vi "DSF Config File to Engine Config Cluster.vi"(8 "error in (no error)":errorcluster, 11 "dsf configuration file path":path) -> (0 "error out":errorcluster, 3 "output cluster":T1)   [LabVIEW 2017, in "Data Sharing Framework Engine.lvlib"]
uses:
  Data Sharing Framework Engine.lvlib
  Configuration/1.0.0/Public/Controls/DSF Engine Framework Configuration.ctl
  Configuration/1.0.0/Public/Controls/DSF Engine Plugin Configuration.ctl
  Configuration/1.0.0/Public/Controls/DSF Timing Info.ctl
  Configuration/1.0.0/Public/Controls/DSF Engine Transfer Group Configuration.ctl
  Configuration/1.0.0/Public/Controls/DSF Direction.ctl
  Configuration/1.0.0/Public/Controls/DSF Engine Transfer Configuration.ctl
  Configuration/1.0.0/Public/Controls/DSF Byte Order.ctl
  Configuration/1.0.0/Public/Controls/DSF Engine Channel Configuration.ctl
  Configuration/1.0.0/Public/Controls/DSF Data Type.ctl
  Configuration/1.0.0/Public/Controls/DSF Settings Info.ctl
  Configuration/1.0.0/Public/Read All Item IDs/Read All Plugin IDs.vi
  Configuration/1.0.0/Public/Read Item/Read Plugin.vi
  Configuration/1.0.0/Public/Read Item/Read Settings.vi
  Configuration/1.0.0/Public/Read Item/Read Group.vi
  Configuration/1.0.0/Public/Read Item/Read Transfer.vi
  Configuration/1.0.0/Public/Read Item/Read Channel.vi
  Configuration/1.0.0/Data Sharing Framework Configuration.lvlib
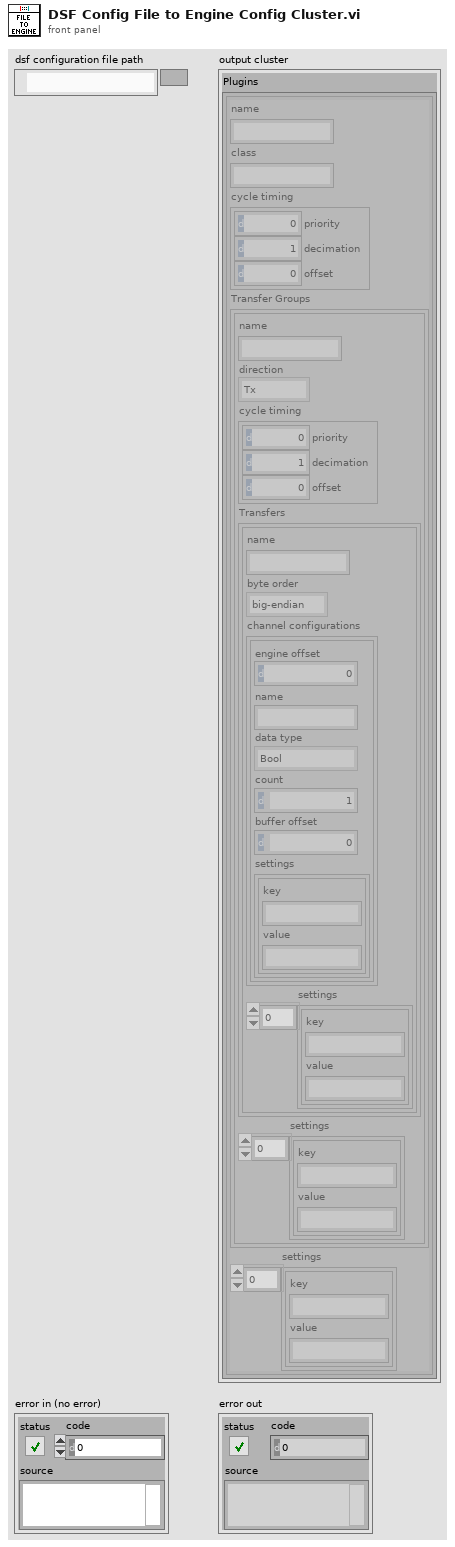
[diagram p1: front panel]
types:
  T1 = typedef "Data Sharing Framework Configuration.lvlib/DSF Engine Framework Configuration.ctl" = cluster{"Plugins":T2[]}
  T2 = typedef "Data Sharing Framework Configuration.lvlib/DSF Engine Plugin Configuration.ctl" = cluster{"name":string, "class":string, "cycle timing":T3, "Transfer Groups":T4[], "settings":T10}
  T3 = typedef "Data Sharing Framework Configuration.lvlib/DSF Timing Info.ctl" = cluster{"priority":u64, "decimation":u64, "offset":u64}
  T4 = typedef "Data Sharing Framework Configuration.lvlib/DSF Engine Transfer Group Configuration.ctl" = cluster{"name":string, "direction":T5, "cycle timing":T3, "Transfers":T6[], "settings":T10}
  T5 = typedef "Data Sharing Framework Configuration.lvlib/DSF Direction.ctl" = enum8{"Tx", "Rx"}
  T6 = typedef "Data Sharing Framework Configuration.lvlib/DSF Engine Transfer Configuration.ctl" = cluster{"name":string, "byte order":T7, "channel configurations":T8[], "settings":T10}
  T7 = typedef "Data Sharing Framework Configuration.lvlib/DSF Byte Order.ctl" = enum8{"big-endian", "little-endian"}
  T8 = typedef "Data Sharing Framework Configuration.lvlib/DSF Engine Channel Configuration.ctl" = cluster{"engine offset":u64, "name":string, "data type":T9, "count":u64, "buffer offset":u64, "settings":T10}
  T9 = typedef "Data Sharing Framework Configuration.lvlib/DSF Data Type.ctl" = enum8{"Bool", "SGL", "DBL", "I8", "I16", "I32", "I64", "U8", "U16", "U32", "U64"}
  T10 = typedef "Data Sharing Framework Configuration.lvlib/DSF Settings Info.ctl" = cluster{"key":string, "value":string}[]
  T11 = typedef "Data Sharing Framework Configuration.lvlib/DSF Config Data RefNum.ctl" = refnum<k1>
  T12 = typedef "Data Sharing Framework Configuration.lvlib/DSF Plugin Info.ctl" = cluster{"type":string, "timing":T3, "group ids":string[], "settings id":string}
  T13 = typedef "Data Sharing Framework Configuration.lvlib/DSF Group Info.ctl" = cluster{"direction":T5, "timing":T3, "transfer ids":string[], "settings id":string}
  T14 = typedef "Data Sharing Framework Configuration.lvlib/DSF Transfer Info.ctl" = cluster{"byte order":T7, "channel ids":string[], "settings id":string}
  T15 = typedef "Data Sharing Framework Configuration.lvlib/DSF Channel Info.ctl" = cluster{"count":u64, "buffer offset":u64, "data type":T9, "settings id":string}
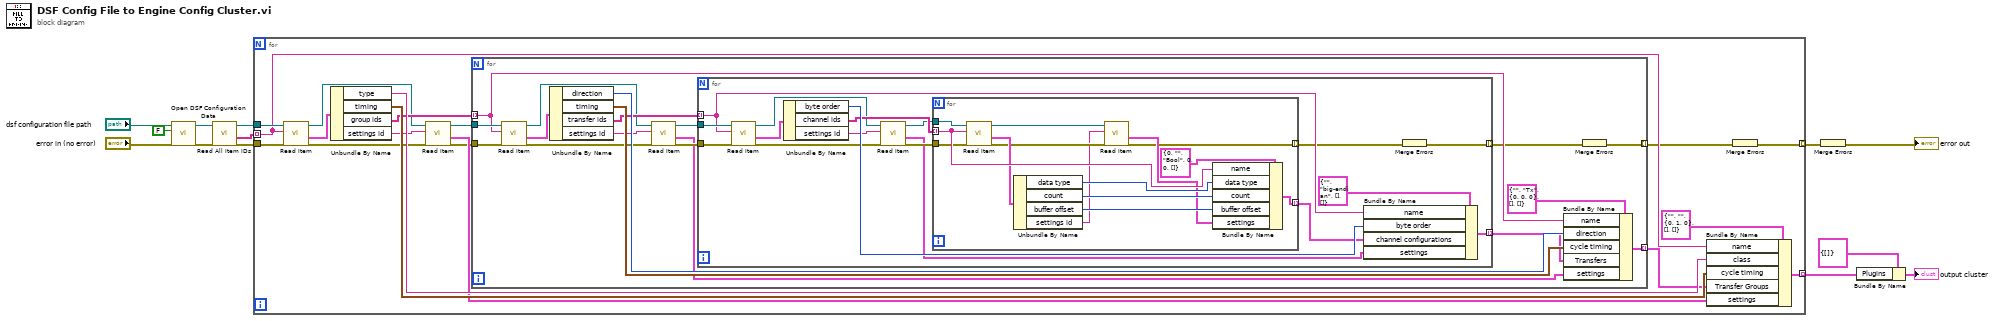
[diagram p0: block diagram]
diagram:
  n1 = call "Open DSF Configuration Data.vi"("error in (no error)"="error in (no error)", "create file if necessary (T)"=FALSE, "dsf configuration file path"="dsf configuration file path") -> ("error out"=w10:errorcluster, "dsf refnum"=w11:T11)  [unwired: 4 in, 3 out]
  n2 = call-poly "Read All Item IDs.vi"("error in (no error)"=w10, "dsf refnum"=w11) -> ("error out"=w6:errorcluster, "Plugin IDs"=w8:string[], "dsf refnum out"=w7:T11)  [unwired: 7 in]
  n3 = for {
    tunnel: w8 -> [w23] mode=indexing
    tunnel: w7 -> [w30]
    tunnel: [w26] -> w2 mode=indexing
    tunnel: w6 -> [w17]
    tunnel: [w14] -> w5 mode=indexing
    n4 = call-poly "Read Item.vi"("error in (no error)"=w17, "Plugin ID"=w23, "dsf refnum"=w30) -> ("error out"=w18:errorcluster, "value"=w29:T12, "dsf refnum out"=w22:T11)  [unwired: 5 in, 1 out]
    n5 = Unbundle By Name(w29) -> ("type"=w28:string, "timing"=w27:T3, "group ids"=w25:string[], "settings id"=w20:string)
    n6 = call-poly "Read Item.vi"("error in (no error)"=w18, "Settings ID"=w20, "dsf refnum"=w22) -> ("error out"=w16:errorcluster, "value"=w19:T10, "dsf refnum out"=w21:T11)  [unwired: 5 in, 1 out]
    n7 = for {
      tunnel: w21 -> [w49]
      tunnel: w25 -> [w46] mode=indexing
      tunnel: [w43] -> w24 mode=indexing
      tunnel: w16 -> [w40]
      tunnel: [w32] -> w15 mode=indexing
      n8 = call-poly "Read Item.vi"("error in (no error)"=w40, "Group ID"=w46, "dsf refnum"=w49) -> ("error out"=w36:errorcluster, "value"=w47:T13, "dsf refnum out"=w39:T11)  [unwired: 5 in, 1 out]
      n9 = Unbundle By Name(w47) -> ("direction"=w45:T5, "timing"=w44:T3, "transfer ids"=w42:string[], "settings id"=w37:string)
      n10 = call-poly "Read Item.vi"("error in (no error)"=w36, "Settings ID"=w37, "dsf refnum"=w39) -> ("error out"=w35:errorcluster, "value"=w34:T10, "dsf refnum out"=w38:T11)  [unwired: 5 in, 1 out]
      n11 = for {
        tunnel: w42 -> [w59] mode=indexing
        tunnel: w38 -> [w66]
        tunnel: [w63] -> w41 mode=indexing
        tunnel: w35 -> [w58]
        tunnel: [w51] -> w33 mode=indexing
        n12 = call-poly "Read Item.vi"("error in (no error)"=w58, "Transfer ID"=w59, "dsf refnum"=w66) -> ("error out"=w56:errorcluster, "value"=w65:T14, "dsf refnum out"=w60:T11)  [unwired: 5 in, 1 out]
        n13 = Unbundle By Name(w65) -> ("byte order"=w64:T7, "channel ids"=w61:string[], "settings id"=w55:string)
        n14 = call-poly "Read Item.vi"("error in (no error)"=w56, "Settings ID"=w55, "dsf refnum"=w60) -> ("error out"=w54:errorcluster, "value"=w53:T10, "dsf refnum out"=w57:T11)  [unwired: 5 in, 1 out]
        n15 = for {
          tunnel: [w80] -> w62 mode=indexing
          tunnel: w61 -> [w78] mode=indexing
          tunnel: w57 -> [w79]
          tunnel: w54 -> [w73]
          tunnel: [w68] -> w52 mode=indexing
          n16 = call-poly "Read Item.vi"("error in (no error)"=w73, "Channel ID"=w78, "dsf refnum"=w79) -> ("error out"=w71:errorcluster, "value"=w77:T15, "dsf refnum out"=w72:T11)  [unwired: 5 in, 1 out]
          n17 = Unbundle By Name(w77) -> ("data type"=w76:T9, "count"=w75:u64, "buffer offset"=w74:u64, "settings id"=w70:string)
          n18 = call-poly "Read Item.vi"("error in (no error)"=w71, "Settings ID"=w70, "dsf refnum"=w72) -> ("error out"=w68:errorcluster, "value"=w69:T10)  [unwired: 5 in, 2 out]
          n19 = Bundle By Name(cluster=T8 {"engine offset"=0, "name"="", "data type"=enum."Bool", "count"=0, "buffer offset"=0, "settings"=[]} ("channel configurations"), "name"=w78, "data type"=w76, "count"=w75, "buffer offset"=w74, "settings"=w69) -> (w80:T8)
        }
        n20 = Bundle By Name(cluster=T6 {"name"="", "byte order"=enum."big-endian", "channel configurations"=[], "settings"=[]} ("Transfer Configuration"), "name"=w59, "byte order"=w64, "channel configurations"=w62, "settings"=w53) -> (w63:T6)
        n21 = Merge Errors(w52) -> (w51:errorcluster)
      }
      n22 = Bundle By Name(cluster=T4 {"name"="", "direction"=enum."Tx", "cycle timing"={"priority"=0, "decimation"=0, "offset"=0}, "Transfers"=[], "settings"=[]} ("Transfer Group Configuration"), "name"=w46, "direction"=w45, "cycle timing"=w44, "Transfers"=w41, "settings"=w34) -> (w43:T4)
      n23 = Merge Errors(w33) -> (w32:errorcluster)
    }
    n24 = Bundle By Name(cluster=T2 {"name"="", "class"="", "cycle timing"={"priority"=0, "decimation"=1, "offset"=0}, "Transfer Groups"=[], "settings"=[]} ("Plugin Configuration"), "name"=w23, "class"=w28, "cycle timing"=w27, "Transfer Groups"=w24, "settings"=w19) -> (w26:T2)
    n25 = Merge Errors(w15) -> (w14:errorcluster)
  }
  n26 = Merge Errors(w5) -> (→"error out":errorcluster)
  n27 = Bundle By Name(cluster=T1 {"Plugins"=[]} ("Framework Config (JSON)"), "Plugins"=w2) -> (→"output cluster":T1)
